vi "Variable_local.vi"() -> ()   [LabVIEW 2017]
panel:
  in  "milliseconds to wait 2":u32
  out "Waveform Chart 2":dbl(graph)
  in  "Stop Button 2":bool
  in  "Stop Button":bool
  out "Waveform Chart":dbl(graph)
  in  "milliseconds to wait":u32
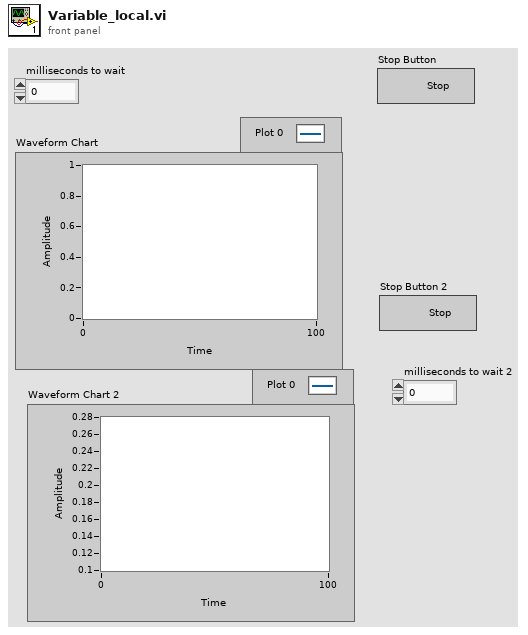
[diagram p1: front panel]
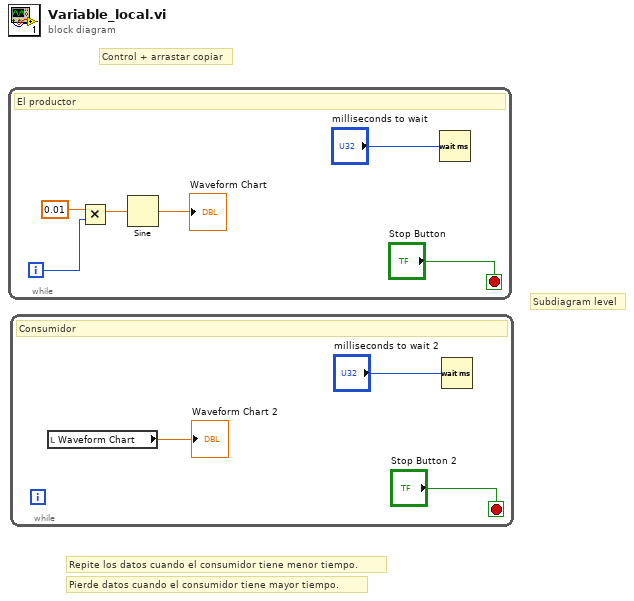
[diagram p0: block diagram]
diagram:
  # "Pierde datos cuando el consumidor tiene mayor tiempo."
  # "Repite los datos cuando el consumidor tiene menor tiempo."
  # "Subdiagram level"
  # "Control + arrastar copiar"
  n1 = while {
    i -> [w4]
    stop <- "Stop Button" stop-if-true
    # "El productor"
    n2 = Multiply(x=0.01, y=w4) -> (x*y=w3:dbl)
    n3 = Sine(x=w3) -> (sin(x)=→"Waveform Chart":dbl)
    n4 = Wait (ms)(milliseconds to wait="milliseconds to wait") -> ()  [unwired: 1 out]
  }
  n5 = while {
    stop <- "Stop Button 2" stop-if-true
    # "Consumidor"
    n6 = local read "Waveform Chart"() -> (→"Waveform Chart 2":dbl)
    n7 = Wait (ms)(milliseconds to wait="milliseconds to wait 2") -> ()  [unwired: 1 out]
  }
